vi "Do Init Teams Array.vi"(6 "Position":T1, 7 "Teams in":refnum<class "Team.lvclass">[](array[class]), 8 "Board Size":i32, 9 "Round":u32, 10 "Team":i32, 11 "Square in":refnum<class "Square.lvclass">) -> (3 "Square out":refnum<class "Square.lvclass">, 5 "Teams out":refnum<class "Team.lvclass">[](array[class]))   [LabVIEW 2020, in "SquareBattle.lvlib" / "Square.lvclass"]
uses:
  Square.lvclass
  Square.lvclass/Square.ctl
  Team/Team.lvclass
  Position.ctl
  SquareBattle.lvlib
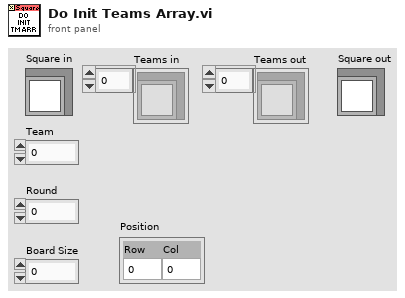
[diagram p1: front panel]
types:
  T1 = typedef "SquareBattle.lvlib/Position.ctl" = cluster{"Row":i32, "Col":i32}
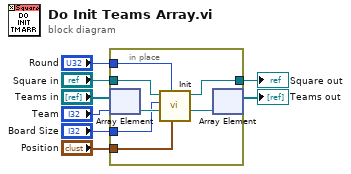
[diagram p0: block diagram]
diagram:
  n1 = in-place {
    in-place-border: "Square in" -> [w14]
    in-place-border: [w13] -> w5
    in-place-border: "Board Size" -> [w11]
    in-place-border: "Position" -> [w10]
    in-place-border: "Round" -> [w9]
    n2 = in-place-array #1("Teams in", "Team") -> (w15:refnum<class "Team.lvclass">)
    n3 = call "Init.vi"("Position"=w10, "Round"=w9, "Team in"=w15, "Board Size"=w11, "Square in"=w14) -> ("Team out"=w12:refnum<class "Team.lvclass">, "Square out"=w13:refnum<class "Square.lvclass">)  [unwired: 5 in]
    n4 = in-place-array #1(w12) -> (→"Teams out":refnum<class "Team.lvclass">[])  [unwired: 1 out]
  }
  "Square out" <- w5
